vi "Check and Generate Path to lv_proc.vi"(8 "error in (no error)":errorcluster, 11 "dir or path to lv_proc.dll (.)":path) -> (0 "error out":errorcluster, 3 "dup path":path)   [LabVIEW 2013, in "LV Process library.lvlib"]
doc: "Checks input path to lv_proc.dll or directory containing lv_proc.dll. If input empty, generate path from application directory. If not empty and is directory, append \"lv_proc.dll\". If not empty and file, consider it as lv_proc.dll. Checks for existence and generate error if needed.\n\nThis vi is intended to use only inside of the LV Process library.\n\n---\nLV Process works only with lv_proc.dll library, which is part of vipm package or should be delivered together with packed library. Placement of this dll is selected in terminal of Create Process.vi."
uses:
  LV Process library.lvlib
  <vilib>/Utility/error.llb/Error Cluster From Error Code.vi
  <vilib>/ErrorRing/Error Ring.xnode
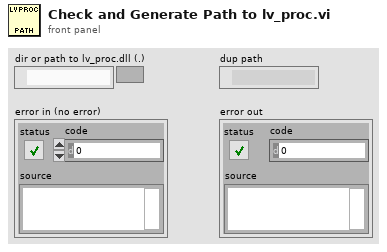
[diagram p1: front panel]
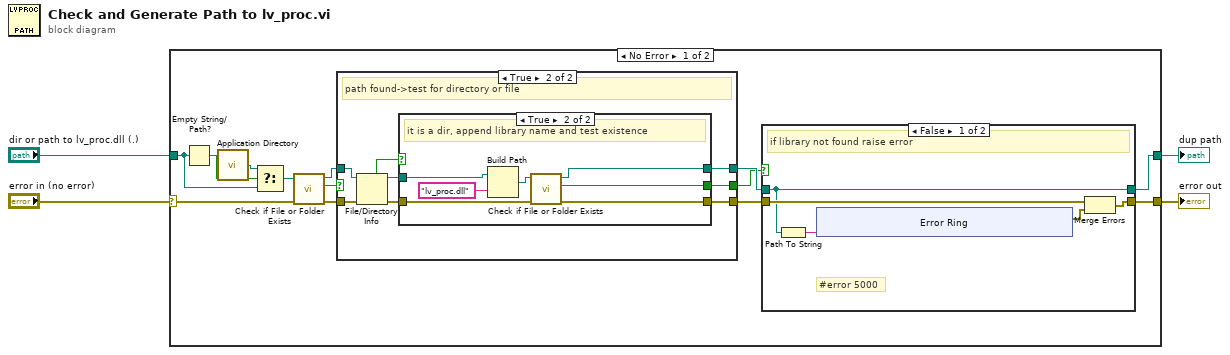
[diagram p0: block diagram]
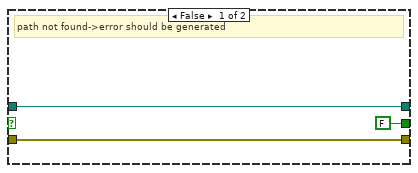
[diagram p3: hidden frame]
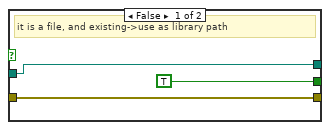
[diagram p4: hidden frame]
diagram:
  n1 = case shown="No Error" "error in (no error)" {
    selector: "error in (no error)" -> [w5 w54]
    tunnel: "dir or path to lv_proc.dll (.)" -> [w11 w53]
    tunnel: [w8 w54] -> w3
    tunnel: [w7 w53] -> w2
    frame No Error {
      n2 = Empty String/Path?(string/path=w11) -> (empty?=w13:bool)
      n3 = call <vilib>:"Application Directory.vi"() -> ("Application Directory"=w12:path)
      n4 = Select(t=w12, s=w13, f=w11) -> (s? t:f=w10:path)
      n5 = call <vilib>:"Check if File or Folder Exists.vi"("error in (no error)"=w5, "path"=w10) -> ("error out"=w6:errorcluster, "file or folder exists?"=w17:bool, "dup path"=w9:path)  [unwired: 7 in]
      n6 = case shown="True" w17 {
        tunnel: w9 -> [w34 w42]
        tunnel: w6 -> [w32 w41]
        tunnel: [w34 w39] -> w16
        tunnel: [FALSE w35] -> w15
        tunnel: [w32 w36] -> w14
        frame False {
          # "path not found->error should be generated"
        }
        frame True {
          # "path found->test for directory or file"
          n7 = File/Directory Info(path=w42, error in=w41) -> (path out=w38:path, directory=w40:bool, error out=w37:errorcluster)  [unwired: 4 out]
          n8 = case shown="True" w40 {
            tunnel: [w45 w46] -> w39
            tunnel: w38 -> [w45 w47]
            tunnel: w37 -> [w43 w50]
            tunnel: [w43 w48] -> w36
            tunnel: [TRUE w49] -> w35
            frame False {
              # "it is a file, and existing->use as library path"
            }
            frame True {
              # "it is a dir, append library name and test existence"
              n9 = Build Path(base path=w47, name or relative path="lv_proc.dll" ("string")) -> (appended path=w51:path)
              n10 = call <vilib>:"Check if File or Folder Exists.vi"("error in (no error)"=w50, "path"=w51) -> ("error out"=w48:errorcluster, "file or folder exists?"=w49:bool, "dup path"=w46:path)  [unwired: 7 in]
            }
          }
        }
      }
      n11 = case shown="False" w15 {
        tunnel: w14 -> [w21 w31]
        tunnel: [w20 w31] -> w8
        tunnel: [w18 w30] -> w7
        tunnel: w16 -> [w18 w30]
        frame False {
          # "#error 5000"
          # "if library not found raise error"
          n12 = Path To String(path=w18) -> (string=w19:string)
          n13 = xnode "Error Ring"("parameter 0"=w19) -> ("error out"=w22:errorcluster)
          n14 = Merge Errors(w21, w22) -> (w20:errorcluster)
        }
        frame True {
          # "all ok"
        }
      }
    }
    frame Error {
    }
  }
  "error out" <- w3
  "dup path" <- w2
